vi "VI Tester About.vi"() -> ()   [LabVIEW 2013, in "GraphicalTestRunner.lvlib"]
uses:
  GraphicalTestRunner.lvlib
panel:
  out "Status":string
  out "Version":string
  in  "Website Button":bool
  out "Social Call to Action":string="Follow us" caption="http://jkisoft.com/tortoisesvn-tool/copyrights/"
  in  "LinkedIn Button":bool caption="http://linkedin.com/company/1161006"
  in  "Twitter Button":bool caption="http://twitter.com/jkisoftware"
  in  "Facebook Button":bool caption="http://facebook.com/JKISoftware"
  in  "Blog Button":bool caption="http://blog.jki.net"
  in  "copyrights":bool
  in  "Cancel":bool
  # "VI Tester for LabVIEW"
  # "© 2007 - 2019 JKI. All Rights Reserved."
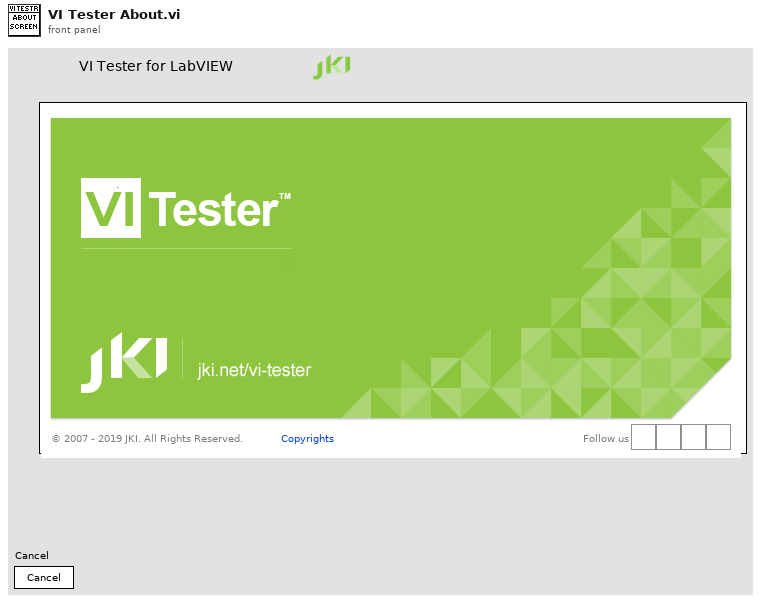
[diagram p1: front panel]
types:
  T1 = enum32{"Invalid", "Default", "Floating", "Floating/Auto-Hide", "Modal"}
  T2 = cluster{"Version":string, "Build Number":u32, "Build Date/Time":dbl}
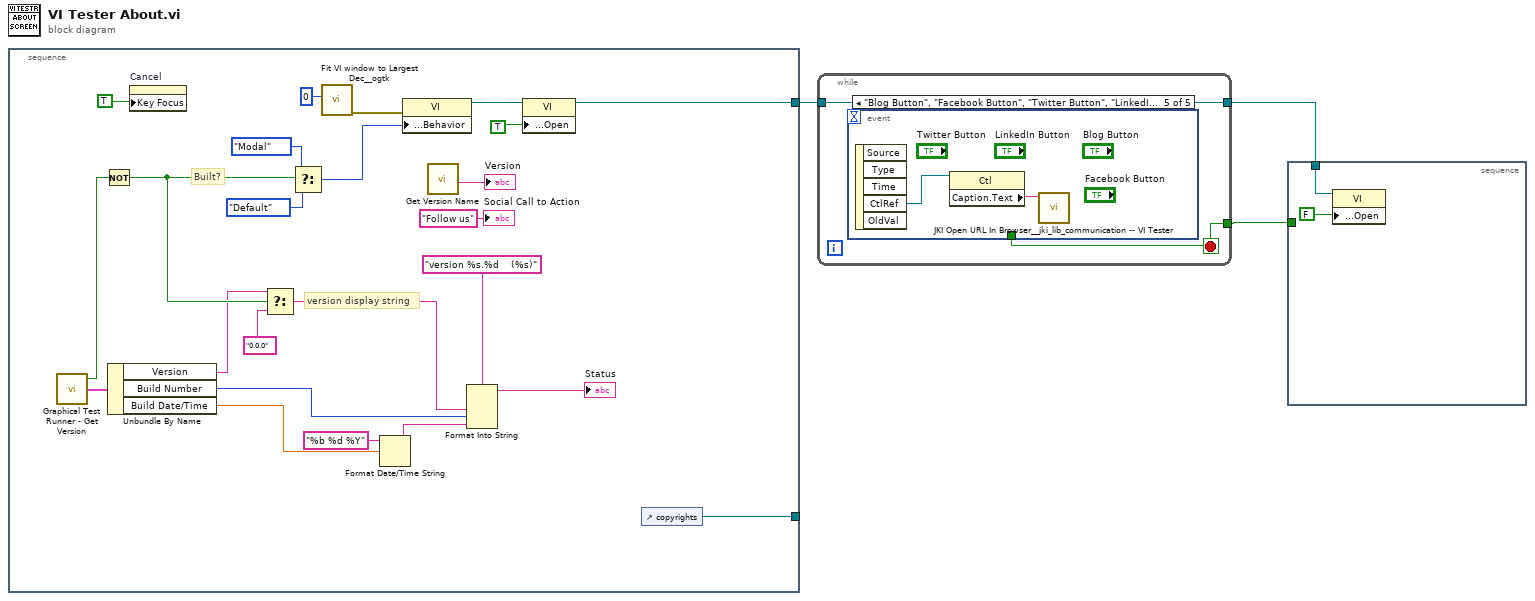
[diagram p0: block diagram]
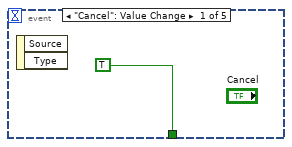
[diagram p2: hidden frame]
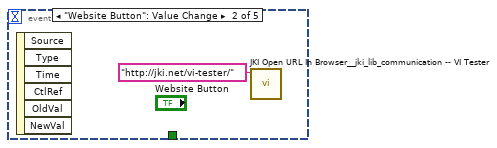
[diagram p3: hidden frame]
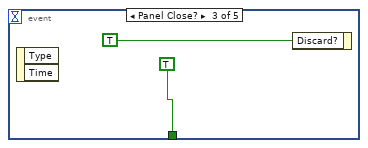
[diagram p4: hidden frame]
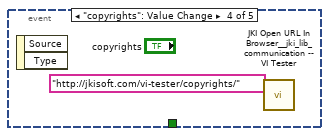
[diagram p5: hidden frame]
diagram:
  n1 = stacked-sequence {
    tunnel: [w7] -> w2
    tunnel: [w9] -> _
    frame #0 {
      # "Built?"
      # "version display string"
      n2 = call "Graphical Test Runner - Get Version.vi"() -> ("Version Info"=w25:T2, "Dev. Environment?"=w16:bool)  [unwired: 4 in]
      n3 = Not(x=w16) -> (.not. x?=w15:bool)
      n4 = Unbundle By Name(w25) -> ("Version"=w14:string, "Build Number"=w20:u32, "Build Date/Time"=w21:dbl)
      n5 = property on="Cancel" class="Bool"("Key Focus"=TRUE) -> ()  [unwired: 2 in, 2 out]
      n6 = Select(t=w14, s=w15, f="0.0.0") -> (s? t:f=w13:string)
      n7 = Select(t=T1."Modal" ("Front Panel Window:Behavior"), s=w15, f=T1."Default" ("Front Panel Window:Behavior")) -> (s? t:f=w17:T1)
      n8 = call <userlib>:"Fit VI window to Largest Dec__ogtk.vi"("border spacing (2 px)"=0) -> ("error out"=w11:errorcluster)  [unwired: 5 in, 1 out]
      n9 = Format Date/Time String(time format string (%c)="%b %d %Y", seconds (now)=w21) -> (date/time string=w22:string)  [unwired: 1 in]
      n10 = property class="VI"(error in=w11, "Front Panel Window:Behavior"=w17) -> (reference out=w8:refnum<vi>)  [unwired: 1 in, 1 out]
      n11 = call "Get Version Name.vi"() -> ("Version Name"=→"Version":string)
      n12 = Format Into String(format string="version %s.%d    (%s)", w13, w20, w22) -> (resulting string=→"Status":string)  [unwired: 2 in, 1 out]
      n13 = property class="VI"(reference=w8, "Front Panel.Open"=TRUE ("Front Panel Window:Open")) -> (reference out=w7:refnum<vi>)  [unwired: 1 in, 1 out]
      n14 = control-ref of="copyrights"() -> (w9:refnum<vi>)
      "Social Call to Action" <- "Follow us" ("Social Call to Action")
    }
  }
  n15 = while {
    tunnel: [w29] -> w3
    tunnel: w2 -> [w28]
    tunnel: [w28] -> w1
    stop <- w29 stop-if-true
    n16 = event shown="[4] \"Blog Button\", \"Facebook Button\", \"Twitter Button\", \"LinkedIn Button\", \"Social Call to Action\": Value Change" {
      selector: _ -> [_ _ _ _ _]
      dyn-events: _ -> [_ _ _ _ _]
      timeout: _ -> [_ _ _ _ _]
      tunnel: [TRUE _ TRUE _ _] -> w29
      event "Cancel": Value Change {
        n17 = event-data() -> ()  [unwired: 1 in, 2 out]
      }
      event "Website Button": Value Change {
        n18 = event-data() -> ()  [unwired: 1 in, 6 out]
        n19 = call "JKI Open URL In Browser__jki_lib_communication -- VI Tester.vi"("url"="http://jki.net/vi-tester/") -> ()  [unwired: 5 in, 2 out]
      }
      event Panel Close? {
        n20 = event-data() -> ()  [unwired: 1 in, 2 out]
        n21 = event-data("Discard?"=TRUE) -> ()  [unwired: 1 in, 1 out]
      }
      event "copyrights": Value Change {
        n22 = event-data() -> ()  [unwired: 1 in, 2 out]
        n23 = call "JKI Open URL In Browser__jki_lib_communication -- VI Tester.vi"("url"="http://jkisoft.com/vi-tester/copyrights/") -> ()  [unwired: 5 in, 2 out]
      }
      event "Blog Button", "Facebook Button", "Twitter Button", "LinkedIn Button", "Social Call to Action": Value Change {
        n24 = event-data() -> ("CtlRef"=w36:refnum<vi>)  [unwired: 1 in, 4 out]
        n25 = property class="Ctl"(reference=w36) -> ("Caption.Text"=w35:string)  [unwired: 1 in, 2 out]
        n26 = call "JKI Open URL In Browser__jki_lib_communication -- VI Tester.vi"("url"=w35) -> ()  [unwired: 5 in, 2 out]
      }
    }
  }
  n27 = stacked-sequence {
    tunnel: w3 -> [_]
    tunnel: w1 -> [w37]
    frame #0 {
      n28 = property class="VI"(reference=w37, "Front Panel.Open"=FALSE ("Front Panel Window:Open")) -> ()  [unwired: 1 in, 2 out]
    }
  }
